vi "_Copy 1.vi"(0 "XRef":T5, 1 "State In":T1) -> (14 "Reply":T3, 15 "Fatal Error Out":T2, 16 "State Out":T1)   [LabVIEW 2014, in "Browse_NEVSTOP-LAB.xnode"]
uses:
  Browse_NEVSTOP-LAB.xnode
  <vilib>/XNodeSupport/XNodeXNodeRef.ctl
  _State 1.ctl
  <vilib>/XNodeSupport/XNodeStringArray.ctl
  <vilib>/XNodeSupport/XNodeString.ctl
  <vilib>/XNodeSupport/XNodeErrorCluster.ctl
  <vilib>/XNodeSupport/NI_XNodeSupport.lvlib
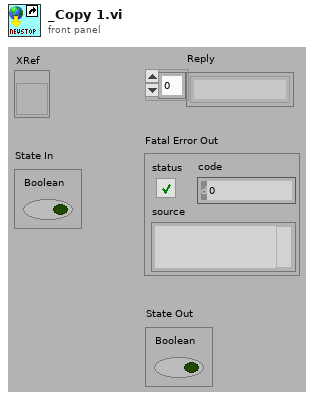
[diagram p1: front panel]
types:
  T1 = typedef "Browse_NEVSTOP-LAB.xnode/_State 1.ctl" = cluster{"Boolean":bool}
  T2 = typedef "NI_XNodeSupport.lvlib/XNodeErrorCluster.ctl" = errorcluster
  T3 = typedef "NI_XNodeSupport.lvlib/XNodeStringArray.ctl" = T4[]
  T4 = typedef "NI_XNodeSupport.lvlib/XNodeString.ctl" = string
  T5 = typedef "NI_XNodeSupport.lvlib/XNodeXNodeRef.ctl" = refnum<vi>
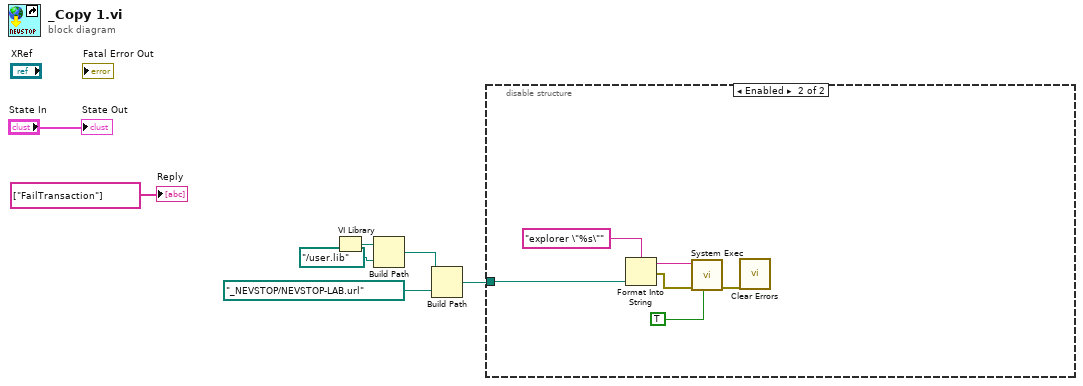
[diagram p0: block diagram]
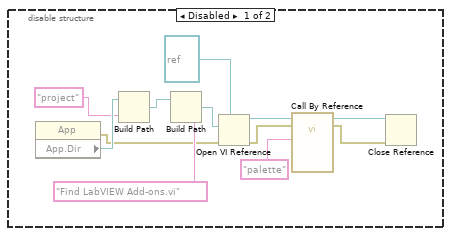
[diagram p2: hidden frame]
diagram:
  n1 = VI Library() -> (path=w2:path)
  n2 = Build Path(base path=w2, name or relative path=path "../user.lib" ("Relative path (.)")) -> (appended path=w3:path)
  n3 = Build Path(base path=w3, name or relative path=path "_NEVSTOP/NEVSTOP-LAB.url" ("Relative path (.)")) -> (appended path=w4:path)
  n4 = disable-structure shown="Enabled" {
    disable-tunnel: w4 -> [_ w25]
    frame Disabled {
      n5 = property class="App"() -> (error out=w14:errorcluster, "App.Dir"=w19:path)  [unwired: 2 in, 1 out]
      n6 = Build Path(base path=w19, name or relative path="project") -> (appended path=w17:path)
      n7 = Build Path(base path=w17, name or relative path="Find LabVIEW Add-ons.vi") -> (appended path=w15:path)
      n8 = Open VI Reference(type specifier VI Refnum (for type only)=refnum<vi> refnum ("reference"), vi path=w15, error in (no error)=w14) -> (vi reference=w12:refnum<vi>, error out=w9:errorcluster)  [unwired: 3 in]
      n9 = call-by-ref "?"(reference=w12, error in=w9, "Source"="palette") -> (reference out=w8:refnum<vi>, error out=w10:errorcluster)  [unwired: 11 in]
      n10 = Close Reference(reference=w8, error in (no error)=w10) -> ()  [unwired: 1 out]
    }
    frame Enabled {
      n11 = Format Into String(format string="explorer \"%s\"" ("command line"), w25) -> (resulting string=w23:string, error out=w20:errorcluster)  [unwired: 2 in]
      n12 = call <vilib>:"System Exec.vi"("run minimized? (F)"=TRUE, "error in (no error)"=w20, "command line"=w23) -> ("error out"=w21:errorcluster)  [unwired: 5 in, 3 out]
      n13 = call <vilib>:"Clear Errors.vi"("error in (no error)"=w21) -> ()  [unwired: 5 in, 2 out]
    }
  }
  "Reply" <- T3 ["FailTransaction"] ("Reply")
  "State Out" <- "State In"
